vi "calculateTableSimpleSerpentine.vi"(5 "scan length y":dbl format="%#_13g", 6 "number of times to go over table":i32=1, 7 "steps Y":i32, 8 "scan length x":dbl format="%#_13g", 9 "steps X":i32) -> (0 "stepsize y":dbl, 1 "final array Y":dbl[](array[numeric]), 2 "stepsize x":dbl, 3 "final array X":dbl[](array[numeric]), 4 "size x":i32)   [LabVIEW 2016]
panel:
  out "size y":i32
  out "onescan x":dbl[](array[numeric])
  out "middle x":dbl
  out "onescan x offset":dbl[](array[numeric])
  out "onescan y offset":dbl[](array[numeric])
  out "middle y":dbl
  out "onescan y":dbl[](array[numeric])
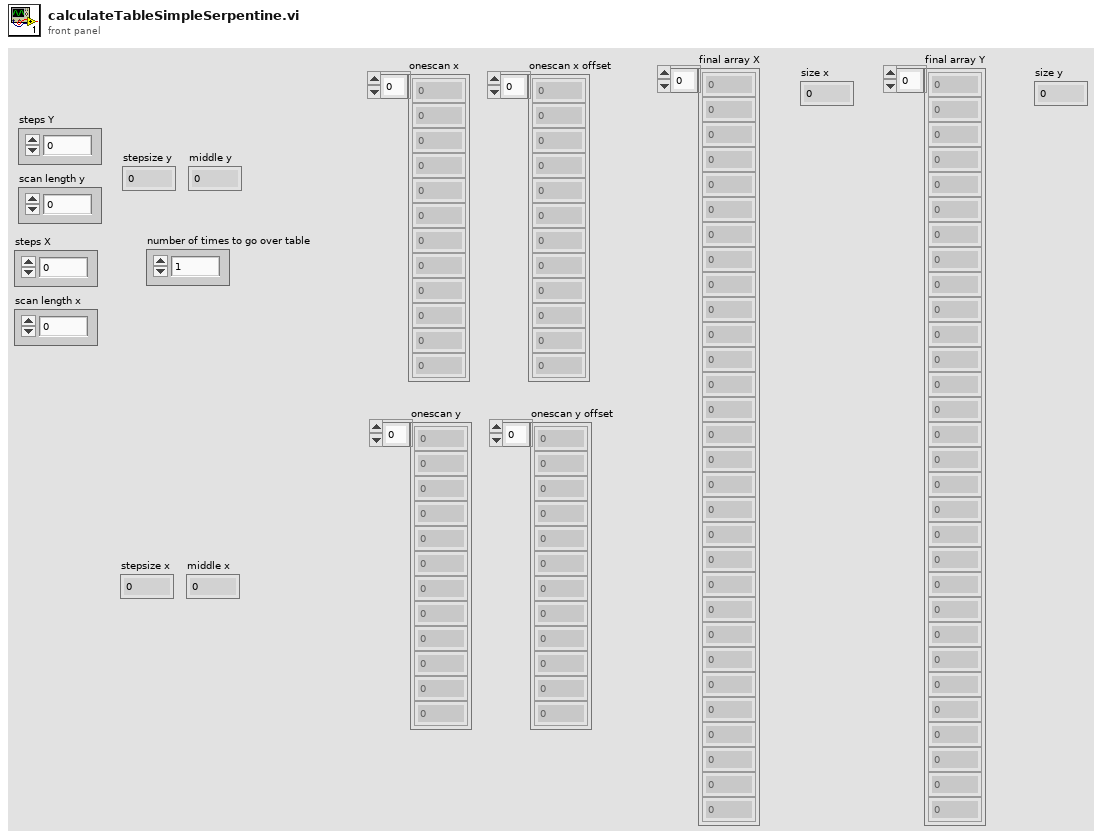
[diagram p1: front panel]
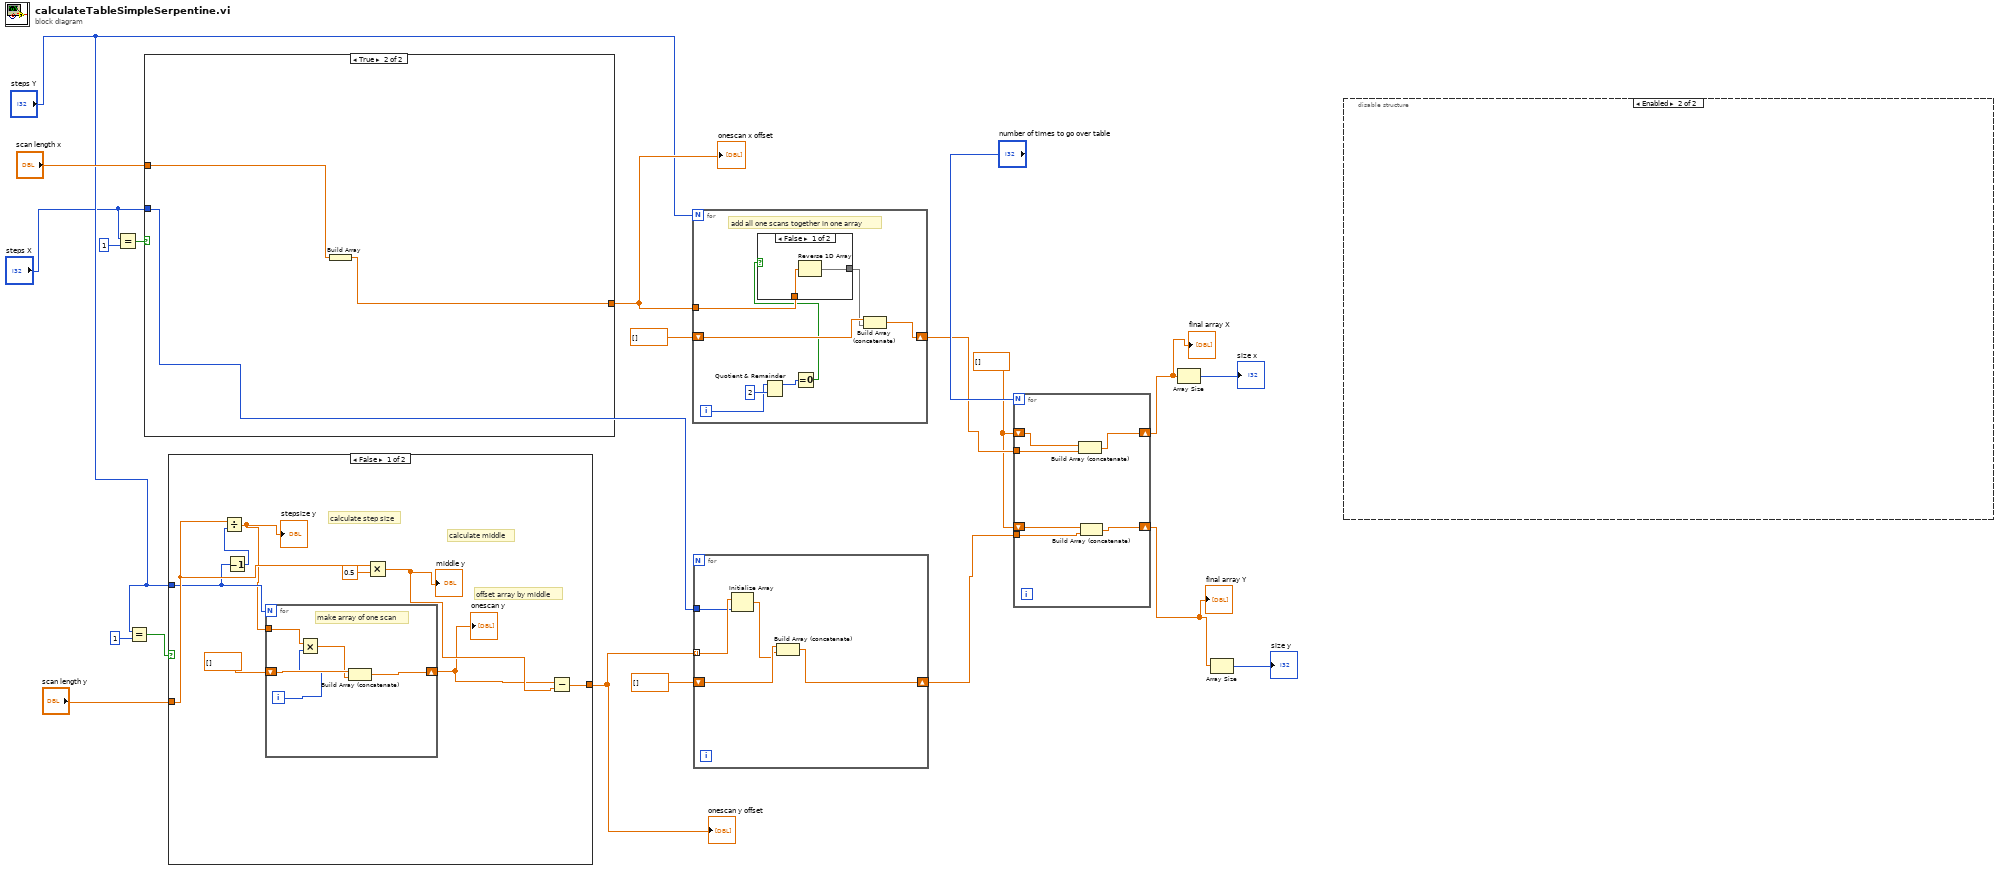
[diagram p0: block diagram]
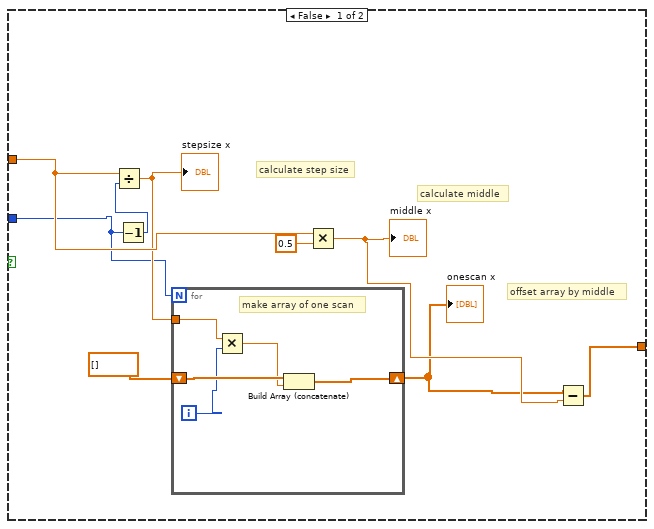
[diagram p2: hidden frame]
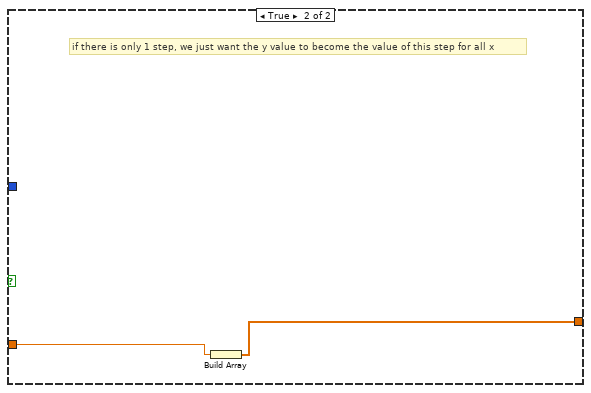
[diagram p3: hidden frame]
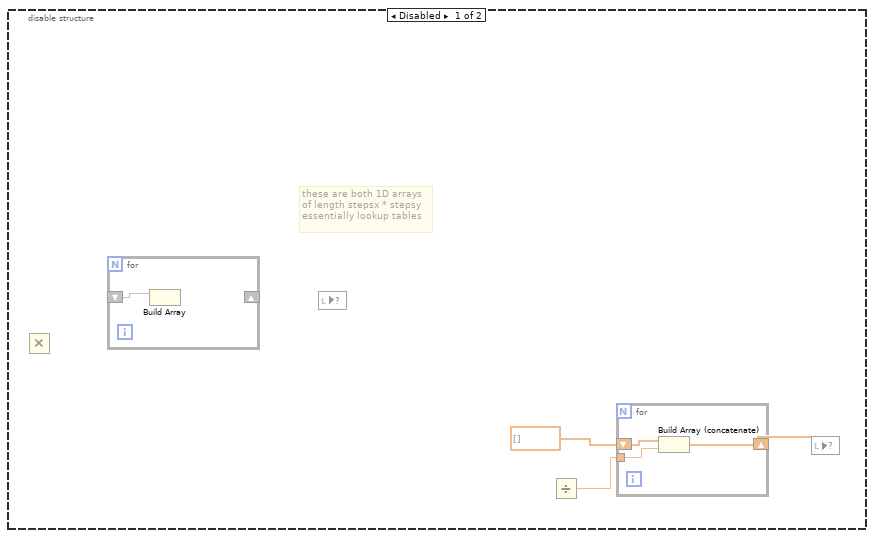
[diagram p5: hidden frame]
diagram:
  w7 = dbl[] []
  n1 = Equal?(x="steps X", y=1) -> (x = y?=w2:bool)
  n2 = Equal?(x="steps Y", y=1) -> (x = y?=w4:bool)
  n3 = case shown="True" w2 {
    tunnel: "scan length x" -> [w26 w35]
    tunnel: [w22 w36] -> w16
    tunnel: "steps X" -> [w21 _]
    frame False {
      # "calculate middle"
      # "offset array by middle"
      # "calculate step size"
      n4 = Decrement(x=w21) -> (x-1=w28:i32)
      n5 = Divide(x=w26, y=w28) -> (x/y=w25:dbl)
      "stepsize x" <- w25
      n6 = for {
        N: w21 -> [_]
        shift-right: [w33] -> w23
        shift-left: dbl[] [] -> [w34]
        tunnel: w25 -> [w32]
        i -> [w30]
        # "make array of one scan"
        n7 = Multiply(x=w32, y=w30) -> (x*y=w31:dbl)
        n8 = Build Array (concatenate)(w34, w31) -> (w33:dbl[])
      }
      "onescan x" <- w23
      n9 = Multiply(x=w26, y=0.5) -> (x*y=w24:dbl)
      "middle x" <- w24
      n10 = Subtract(x=w23, y=w24) -> (x-y=w22:dbl[])
    }
    frame True {
      n11 = Build Array(w35) -> (w36:dbl[])
    }
  }
  "onescan x offset" <- w16
  n12 = case shown="False" w4 {
    tunnel: "scan length y" -> [w42 w52]
    tunnel: [w39 w51] -> w15
    tunnel: "steps Y" -> [w38 _]
    frame False {
      # "calculate middle"
      # "offset array by middle"
      # "calculate step size"
      n13 = Decrement(x=w38) -> (x-1=w44:i32)
      n14 = Divide(x=w42, y=w44) -> (x/y=w37:dbl)
      "stepsize y" <- w37
      n15 = for {
        N: w38 -> [_]
        shift-right: [w49] -> w40
        shift-left: dbl[] [] -> [w50]
        tunnel: w37 -> [w48]
        i -> [w46]
        # "make array of one scan"
        n16 = Multiply(x=w48, y=w46) -> (x*y=w47:dbl)
        n17 = Build Array (concatenate)(w50, w47) -> (w49:dbl[])
      }
      "onescan y" <- w40
      n18 = Multiply(x=w42, y=0.5) -> (x*y=w41:dbl)
      "middle y" <- w41
      n19 = Subtract(x=w40, y=w41) -> (x-y=w39:dbl[])
    }
    frame True {
      # "if there is only 1 step, we just want the y value to become the value of this step for all x"
      n20 = Build Array(w52) -> (w51:dbl[])
    }
  }
  "onescan y offset" <- w15
  n21 = for {
    N: "steps Y" -> [_]
    tunnel: w16 -> [w56]
    shift-right: [w59] -> w11
    shift-left: dbl[] [] -> [w60]
    i -> [w57]
    # "add all one scans together in one array"
    n22 = Quotient & Remainder(x=w57, y=2) -> (x-y*floor(x/y)=w54:i32)  [unwired: 1 out]
    n23 = Equal To 0?(x=w54) -> (x = 0?=w53:bool)
    n24 = case shown="False" w53 {
      tunnel: w56 -> [w62 w63]
      tunnel: [w61 w63] -> w55
      frame False {
        n25 = Reverse 1D Array(array=w62) -> (reversed array=w61:dbl[])
      }
      frame True {
      }
    }
    n26 = Build Array (concatenate)(w60, w55) -> (w59:dbl[])
  }
  n27 = for {
    tunnel: w15 -> [w66] mode=indexing
    shift-right: [w67] -> w8
    shift-left: dbl[] [] -> [w68]
    tunnel: "steps X" -> [w65]
    n28 = Initialize Array(w66, w65) -> (w64:dbl[])
    n29 = Build Array (concatenate)(w68, w64) -> (w67:dbl[])
  }
  n30 = for {
    N: "number of times to go over table" -> [_]
    shift-right: [w72] -> w10
    shift-left: w7 -> [w74]
    tunnel: w11 -> [w73]
    shift-right: [w70] -> w9
    shift-left: w7 -> [w71]
    tunnel: w8 -> [w69]
    n31 = Build Array (concatenate)(w74, w73) -> (w72:dbl[])
    n32 = Build Array (concatenate)(w71, w69) -> (w70:dbl[])
  }
  "final array Y" <- w9
  "final array X" <- w10
  n33 = Array Size(array=w10) -> (size(s)=→"size x":i32)
  n34 = Array Size(array=w9) -> (size(s)=→"size y":i32)
  n35 = disable-structure shown="Enabled" {
    frame Disabled {
      # "these are both 1D arrays \nof length stepsx * stepsy\nessentially lookup tables"
      n36 = Multiply() -> (y=w75:dbl)  [unwired: 1 in, 1 out]
      n37 = for {
        shift-right: _ -> [_]
        shift-left: _ -> [w80]
        n38 = Build Array(w80) -> ()  [unwired: 1 in, 1 out]
      }
      n39 = local read item#-1() -> ()  [unwired: 1 in]
      n40 = Divide() -> (x=w79:dbl, x/y=w78:dbl)  [unwired: 1 in]
      n41 = for {
        shift-right: [w82] -> w76
        shift-left: dbl[] [] -> [w81]
        tunnel: w78 -> [w83]
        n42 = Build Array (concatenate)(w81, w83) -> (w82:dbl[])
      }
      n43 = local write item#-1(w76) -> ()
    }
    frame Enabled {
    }
  }
